vi "{{Msg}}.vi"(6 "Error":errorcluster, 7 "Actor":refnum<class "Actor.lvclass">, 11 "Message":refnum<class "Msg.lvclass">) -> (3 "Message":refnum<class "Msg.lvclass">, 4 "Error":errorcluster, 5 "Actor":refnum<class "Actor.lvclass">)   [LabVIEW 2020, in "_Template.lvlib" / "{{Actor}}.lvlib" / "Actor.lvclass"]
uses:
  Actor.lvclass
  Actor.lvclass/Actor.ctl
  C:/Users/nathan.davis/Desktop/personal/jettl-harness/repos/jettl/src/jettl Tools/_Template/{{Actor}}/ConcreteActor/Actor.lvclass
  C:/Users/nathan.davis/Desktop/personal/jettl-harness/repos/jettl/src/jettl Tools/_Template/{{Msg}}/ActorMsg/ActorMsg.lvclass
  C:/Users/nathan.davis/Desktop/personal/jettl-harness/repos/jettl/src/jettl/jettl/Actor/Actor.lvclass
  {{Msg}}/{{Msg}}.lvlib
  {{Msg}}/Msg/Msg.lvclass
panel:
  # "This front panel should not be manipulated."
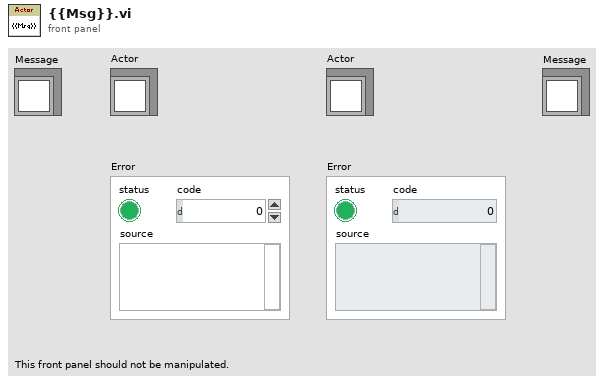
[diagram p1: front panel]
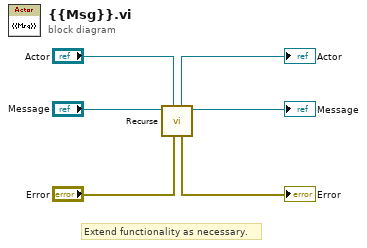
[diagram p0: block diagram]
diagram:
  # "Extend functionality as necessary."
  n1 = call "Recurse.vi"("Error"="Error", "Actor"="Actor", "Msg"="Message") -> ("Msg"=→"Message":refnum<class "Msg.lvclass">, "Error"=→"Error":errorcluster, "Actor"=→"Actor":refnum<class "Actor.lvclass">)  [unwired: 6 in]
